vi "Error Processor.vi"(8 "error in (no error)":errorcluster, 11 "Kasli Wrapper in":refnum<class "Kasli Wrapper 2.0.lvclass">) -> (0 "error out":errorcluster, 3 "Kasli Wrapper out":refnum<class "Kasli Wrapper 2.0.lvclass">)   [LabVIEW 2020, in "Kasli Wrapper 2.0.lvlib" / "Kasli Wrapper 2.0.lvclass"]
doc: "Use this VI to process all the error that are solvable inside this specific uService. Whatever is not possible to process, let it leave this VI and it will be processed by the Error Manager of the Distributed System."
uses:
  Kasli Wrapper 2.0.lvclass
  C:/Users/marco/Documents/GitHub_Lab/TALOS/talos/Father of all uServices/Father of all uServices/Father of all uServices.lvclass
  Kasli Wrapper 2.0 Consumer Case Selector.ctl
  Run Utilities/TypeDefs/Messages/Submit Message.ctl
  Run Utilities/TypeDefs/DAQ Control.ctl
  Run Utilities/Run Instance/Run Instance.lvclass
  Kasli Wrapper 2.0.lvclass/Kasli Wrapper 2.0.ctl
  Father of all uServices/Father of all uServices Messages/Consumer Msg/Consumer Msg.lvclass/Consumer Msg.ctl
  Ancestor/Ancestor/Ancestor.lvclass/Ancestor.ctl
  Father of all uServices/Father of all uServices Messages/Consumer Msg/Send Consumer.vi
  Support VIs/Generate Error.vi
  FGV/Error Memory/Get Error Description.vi
  Support VIs/Get PC name.vi
  Ancestor/Ancestor/Read ID.vi
  Support VIs/Get Class Name.vi
  <vilib>/Utility/error.llb/Clear Errors.vi
  FGV/Error Memory/Error Memory Core.vi
  <vilib>/AdvancedString/Delimited String to 1D String Array.vi
  Support VIs/Circus Root Path.vi
  FGV/Error Memory/Error Crt Lvl checker.vi
  FGV/Error Memory/Error Memory Core.vi/40c8088d-b597-4017-91af-faa98e00292e.vi
  FGV/Error Memory/Error Memory Core.vi/d4a3ab98-063c-4e44-b43d-fbdcfe6c2be2.vi
  Father of all uServices/Father of all uServices/Father of all uServices.lvclass
  C:/Users/marco/Documents/GitHub_Lab/TALOS/builds/Actor Framework PPL/Actor Framework.lvlibp/1abvi3w/vi.lib/ActorFramework/Actor/Actor.lvclass
  builds/Actor Framework PPL/Actor Framework.lvlibp/1abvi3w/vi.lib/ActorFramework/Actor/Read Self Enqueuer.vi
  <userlib>/_OpenG.lib/lvdata/lvdata.llb/Get Strings from Enum__ogtk.vi
  builds/Actor Framework PPL/Actor Framework.lvlibp/1abvi3w/vi.lib/ActorFramework/Message Enqueuer/Enqueue.vi
  Support VIs/Global Memory.vi
  <vilib>/Utility/LVClass/Get LV Class Name.vi
  Support VIs/Is in Packed Library.vi
  Support VIs/TALOS Root path.vi
  Support VIs/Read CSV worksheet.vi
  Support VIs/Global Constants.vi
  <vilib>/Utility/error.llb/General Error Handler.vi
  Support VIs/Error Log.vi
  Father of all uServices/Father of all uServices Messages/Consumer Msg/Consumer Msg.lvclass
  Ancestor/Ancestor/Ancestor.lvclass
  <vilib>/Comparison/Equal/Equal Functor/Equal Functor.lvclass
  Run Utilities/Run Utilities.lvlib
  TALOS.lvlib
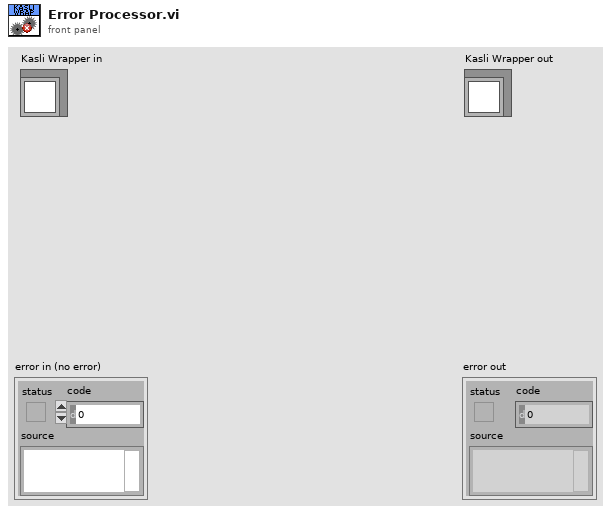
[diagram p1: front panel]
types:
  T1 = typedef "TALOS.lvlib/Run Utilities.lvlib/Submit Message.ctl" = cluster{"DAQ Control":T2, "Run Instance":refnum<class "Run Instance.lvclass">}
  T2 = typedef "TALOS.lvlib/Run Utilities.lvlib/DAQ Control.ctl" = enum16{"On", "Off", "External"}
  T3 = typedef "Kasli Wrapper 2.0.lvlib/Kasli Wrapper 2.0.lvclass/Kasli Wrapper 2.0 Consumer Case Selector.ctl" = enum16{"Init", "Submit Script", "Restart Master", "Master StdOut", "Master StdErr", "Client StdOut", "Client StdErr", "Start Logging", "Stop Logging", "Terminate Script", "Close", "Master ProcessExit"}
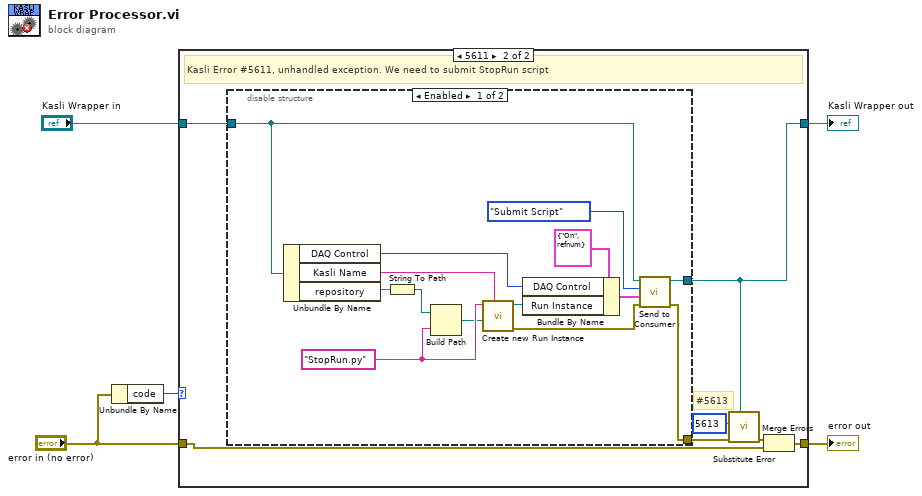
[diagram p0: block diagram]
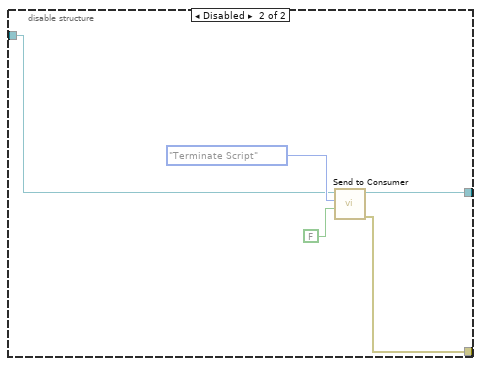
[diagram p3: hidden frame]
diagram:
  n1 = Unbundle By Name("error in (no error)") -> ("code"=w1:i32)
  n2 = case shown="5611" w1 {
    tunnel: "Kasli Wrapper in" -> [w7 w11]
    tunnel: [w7 w12] -> w4
    tunnel: "error in (no error)" -> [w6 w13]
    tunnel: [w6 w14] -> w3
    frame Default {
    }
    frame 5611 {
      # "#5613"
      # "Kasli Error #5611, unhandled exception. We need to submit StopRun script"
      n3 = disable-structure shown="Enabled" {
        disable-tunnel: [w28 w29] -> w12
        disable-tunnel: w11 -> [w27 w31]
        disable-tunnel: [w20 w30] -> w10
        frame Enabled {
          w16 = "StopRun.py" ("string")
          n4 = Unbundle By Name(w27) -> ("DAQ Control"=w24:T2, "Kasli Name"=w19:string, "repository"=w18:string)
          n5 = String To Path(string=w18) -> (path=w17:path)
          n6 = Build Path(base path=w17, name or relative path=w16) -> (appended path=w15:path)
          n7 = call "Create new Run Instance.vi"("Kasli"=w19, "Script Path"=w15, "Script Name"=w16) -> ("error out"=w21:errorcluster, "Run Instance"=w22:refnum<class "Run Instance.lvclass">)  [unwired: 6 in, 1 out]
          n8 = Bundle By Name(cluster=T1 {"DAQ Control"=enum."On", "Run Instance"=refnum} ("Submit Msg"), "DAQ Control"=w24, "Run Instance"=w22) -> (w23:T1)
          n9 = call "Send to Consumer.vi"("error in (no error)"=w21, "Data"=w23, "Case ID"=Kasli_Wrapper_2.0_Consumer_Case_Selector."Submit Script" ("Kasli Wrapper 2 Consumer Case Selector"), "uService Template in"=w27) -> ("error out"=w20:errorcluster, "uService Template out"=w28:refnum<class "Kasli Wrapper 2.0.lvclass">)  [unwired: 6 in]
        }
        frame Disabled {
          n10 = call "Send to Consumer.vi"("Data"=FALSE, "Case ID"=Kasli_Wrapper_2.0_Consumer_Case_Selector."Terminate Script" ("Kasli Wrapper 2 Consumer Case Selector"), "uService Template in"=w31) -> ("error out"=w30:errorcluster, "uService Template out"=w29:refnum<class "Kasli Wrapper 2.0.lvclass">)  [unwired: 7 in]
        }
      }
      n11 = call "Substitute Error.vi"("LabVIEW Object"=w12, "error in (no error)"=w10, "Error Code"=5613) -> ("error out"=w9:errorcluster)  [unwired: 8 in]
      n12 = Merge Errors(w9, w13) -> (w14:errorcluster)
    }
  }
  "error out" <- w3
  "Kasli Wrapper out" <- w4
